vi "Set Current Commands.vi"(8 "error in (no error)":errorcluster, 10 "current commands":dbl[](array[numeric]), 11 "MF3 in":refnum<class "MF3.lvclass">) -> (0 "error out":errorcluster, 3 "MF3 out":refnum<class "MF3.lvclass">)   [LabVIEW 2011, in "MF3.lvclass"]
uses:
  MF3.lvclass
  MF3.lvclass/MF3.ctl
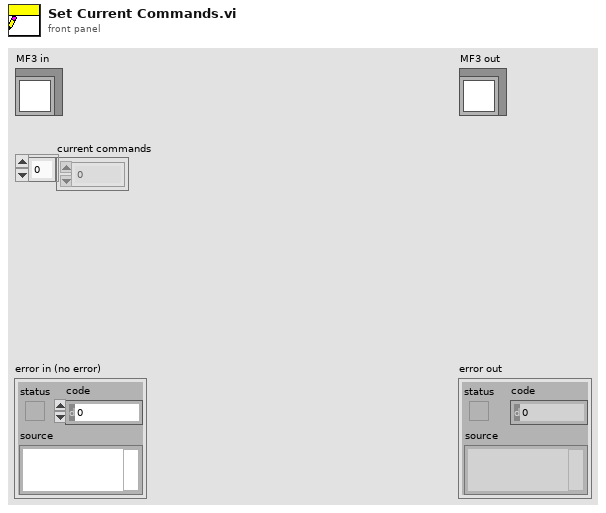
[diagram p1: front panel]
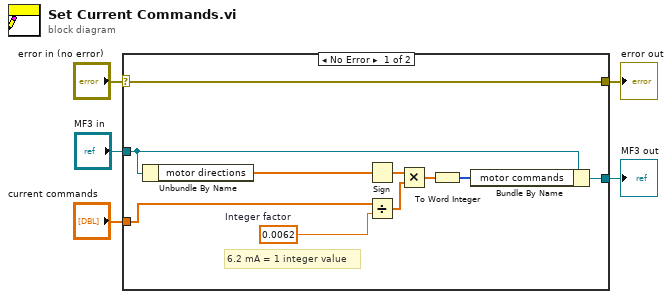
[diagram p0: block diagram]
diagram:
  n1 = case shown="No Error" "error in (no error)" {
    selector: "error in (no error)" -> [w15 w16]
    tunnel: [w15 w16] -> w4
    tunnel: [w14 w17] -> w2
    tunnel: "MF3 in" -> [w10 w17]
    tunnel: "current commands" -> [w12 _]
    frame No Error {
      w13 = 0.0062  # Integer factor
      # "6.2 mA = 1 integer value"
      n2 = Unbundle By Name(w10) -> ("motor directions"=w6:dbl[])
      n3 = Sign(1:w6) -> (0:w7:dbl[])
      n4 = Divide(x=w12, y=w13) -> (x/y=w9:dbl[])
      n5 = Multiply(x=w7, y=w9) -> (x*y=w8:dbl[])
      n6 = To Word Integer(number=w8) -> (16bit integer=w11:i16[])
      n7 = Bundle By Name(cluster=w10, "motor commands"=w11) -> (w14:refnum<class "MF3.lvclass">)
    }
    frame Error {
    }
  }
  "error out" <- w4
  "MF3 out" <- w2
